vi "Find Smallest Circle Value.vi"(7 "Positive ONLY":bool, 10 "Total Circle Value":dbl, 11 "Value":dbl format="%#.6f") -> (3 "Smallest value on the circle":dbl format="%.6f")   [LabVIEW 2023]
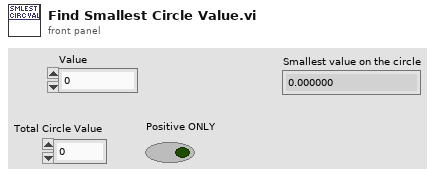
[diagram p1: front panel]
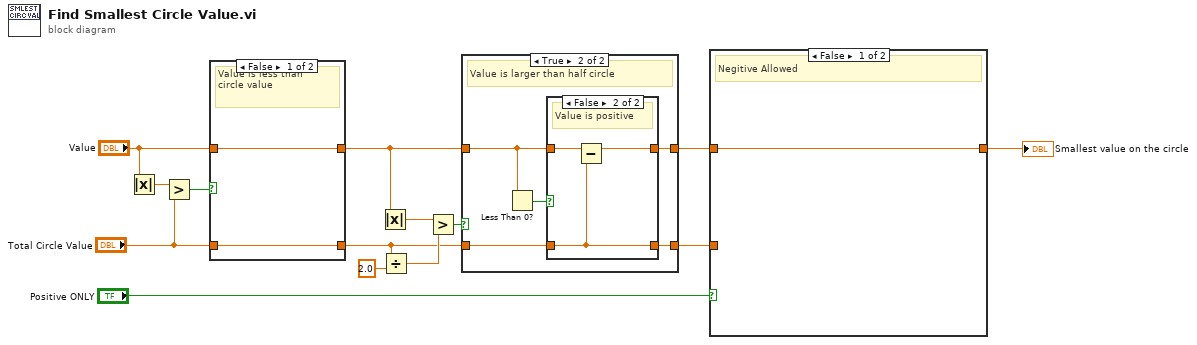
[diagram p0: block diagram]
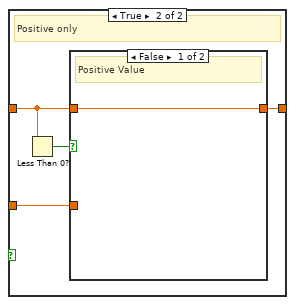
[diagram p2: hidden frame]
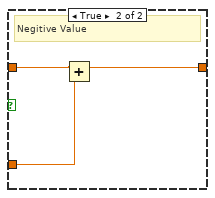
[diagram p3: hidden frame]
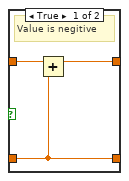
[diagram p5: hidden frame]
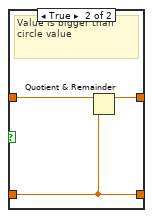
[diagram p6: hidden frame]
diagram:
  n1 = Absolute Value(x="Value") -> (abs(x)=w10:dbl)
  n2 = Greater?(x=w10, y="Total Circle Value") -> (0:w8:bool)
  n3 = case shown="False" w8 {
    tunnel: [w16 w19] -> w6
    tunnel: "Value" -> [w16 w18]
    tunnel: "Total Circle Value" -> [w15 w17]
    tunnel: [w15 w17] -> w5
    frame False {
      # "Value is less than\ncircle value"
    }
    frame True {
      # "Value is bigger than circle value"
      n4 = Quotient & Remainder(x=w18, y=w17) -> (x-y*floor(x/y)=w19:dbl)  [unwired: 1 out]
    }
  }
  n5 = Absolute Value(x=w6) -> (abs(x)=w13:dbl)
  n6 = Divide(x=w5, y=2.0) -> (x/y=w12:dbl)
  n7 = Greater?(x=w13, y=w12) -> (0:w7:bool)
  n8 = case shown="True" w7 {
    tunnel: w6 -> [w21 w25]
    tunnel: w5 -> [w20 w24]
    tunnel: [w21 w23] -> w3
    tunnel: [w20 w22] -> w1
    frame False {
      # "Value is less than half circle"
    }
    frame True {
      # "Value is larger than half circle"
      n9 = Less Than 0?(x=w25) -> (x < 0?=w26:bool)
      n10 = case shown="False" w26 {
        tunnel: w25 -> [w29 w32]
        tunnel: w24 -> [w27 w30]
        tunnel: [w28 w31] -> w23
        tunnel: [w27 w30] -> w22
        frame True {
          # "Value is negitive"
          n11 = Add(x=w29, y=w27) -> (x+y=w28:dbl)
        }
        frame False {
          # "Value is positive"
          n12 = Subtract(x=w32, y=w30) -> (x-y=w31:dbl)
        }
      }
    }
  }
  n13 = case shown="False" "Positive ONLY" {
    tunnel: w3 -> [w33 w36]
    tunnel: [w33 w34] -> w2
    tunnel: w1 -> [_ w35]
    frame False {
      # "Negitive Allowed"
    }
    frame True {
      # "Positive only"
      n14 = Less Than 0?(x=w36) -> (x < 0?=w37:bool)
      n15 = case shown="False" w37 {
        tunnel: w36 -> [w38 w41]
        tunnel: w35 -> [_ w40]
        tunnel: [w38 w39] -> w34
        frame False {
          # "Positive Value"
        }
        frame True {
          # "Negitive Value"
          n16 = Add(x=w41, y=w40) -> (x+y=w39:dbl)
        }
      }
    }
  }
  "Smallest value on the circle" <- w2
